vi "Add Items.vi"(11 "TreeSelection in":refnum<class "TreeSelection.lvclass">) -> (3 "TreeSelection out":refnum<class "TreeSelection.lvclass">)   [LabVIEW 2015, in "TreeControl.lvclass"]
uses:
  TreeControl.lvclass
  TreeSelection/TreeSelection.lvclass
  Add Items Array.ctl
  Add Item Info Cluster.ctl
panel:
  out "Added Tags":string[](array[string])
  in  "Add Items Array":T1
  out "error out":errorcluster
  in  "error in (no error)":errorcluster
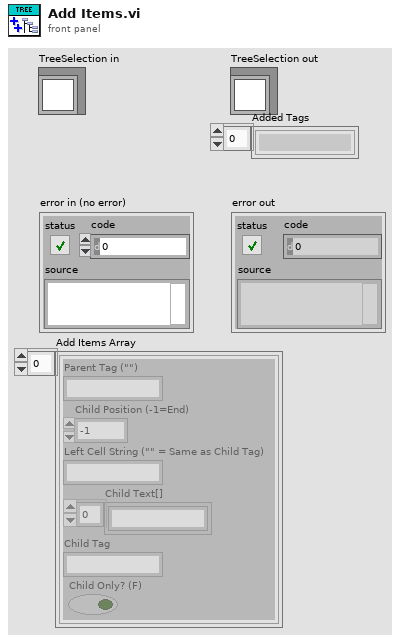
[diagram p1: front panel]
types:
  T1 = typedef "TreeControl.lvclass/Add Items Array.ctl" = T2[]
  T2 = typedef "TreeControl.lvclass/Add Item Info Cluster.ctl" = cluster{"Parent Tag (\"\")":string, "Child Position (-1=End)":i32, "Left Cell String (\"\" = Same as Child Tag)":string, "Child Text[]":string[], "Child Tag":string, "Child Only? (F)":bool}
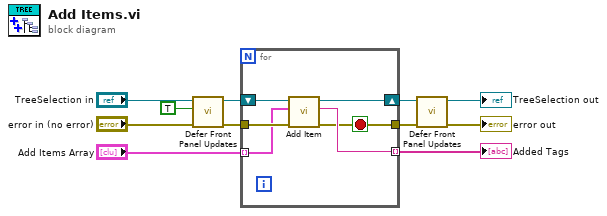
[diagram p0: block diagram]
diagram:
  n1 = call "Defer Front Panel Updates.vi"("error in (no error)"="error in (no error)", "Defer Panel Updates (F)"=TRUE, "Tree in"="TreeSelection in") -> ("error out"=w5:errorcluster, "Tree out"=w11:refnum<class "TreeSelection.lvclass">)  [unwired: 7 in]
  n2 = for {
    shift-right: [w17] -> w9
    shift-left: w11 -> [w16]
    tunnel: w5 -> [w15]
    tunnel: "Add Items Array" -> [w14] mode=indexing
    tunnel: [w13] -> w3 mode=indexing
    tunnel: [w12] -> w2
    stop <- w12 stop-if-true
    n3 = call-dynamic "Add Item.vi"("error in (no error)"=w15, "ItemInfo"=w14, "Tree in"=w16) -> ("error out"=w12:errorcluster, "Add Item Tag"=w13:string, "Tree out"=w17:refnum<class "TreeSelection.lvclass">)  [unwired: 6 in]
  }
  "Added Tags" <- w3
  n4 = call "Defer Front Panel Updates.vi"("error in (no error)"=w2, "Tree in"=w9) -> ("error out"=→"error out":errorcluster, "Tree out"=→"TreeSelection out":refnum<class "TreeSelection.lvclass">)  [unwired: 8 in]
